vi "Get Name.vi"(11 "CD Template":refnum<class "NIVS_CD Template.lvclass">) -> (2 "String":string)   [LabVIEW 2020, in "NIVS_CD Template.lvclass"]
uses:
  NIVS_CD Template.lvclass
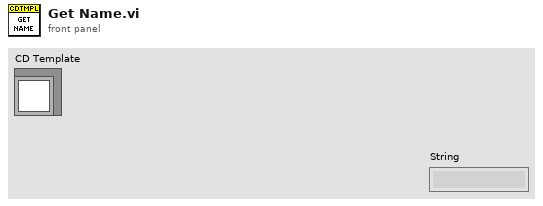
[diagram p1: front panel]
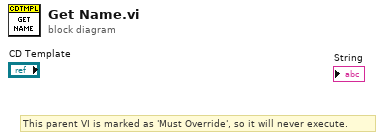
[diagram p0: block diagram]
diagram:
  # "This parent VI is marked as 'Must Override', so it will never execute."
